vi "Init.vi"() -> (3 "xxxxx Msg Strategy out":refnum<class "xxxxx Msg Strategy.lvclass">)   [LabVIEW 2021, in "Providers.lvlib" / "jettl Msg xxxxx.lvlib" / "xxxxx Msg Strategy.lvclass"]
uses:
  xxxxx Msg Strategy.lvclass
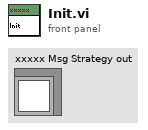
[diagram p1: front panel]
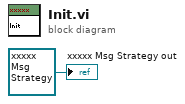
[diagram p0: block diagram]
diagram:
  "xxxxx Msg Strategy out" <- refnum<class "xxxxx Msg Strategy.lvclass"> refnum ("xxxxx Msg Strategy out")
